vi "Update CD Name Constant.vi"(7 "vi Name":string, 8 "error in":errorcluster, 10 "Custom Device Name":string, 11 "lvlib Path":path) -> (0 "error out":errorcluster)   [LabVIEW 2026, in "NIVS_CDEW_MetaDataObj.lvclass"]
uses:
  NIVS_CDEW_MetaDataObj.lvclass
  NIVS_CDEW_MetaDataObj.lvclass/NIVS_CDEW_MetaDataObj.ctl
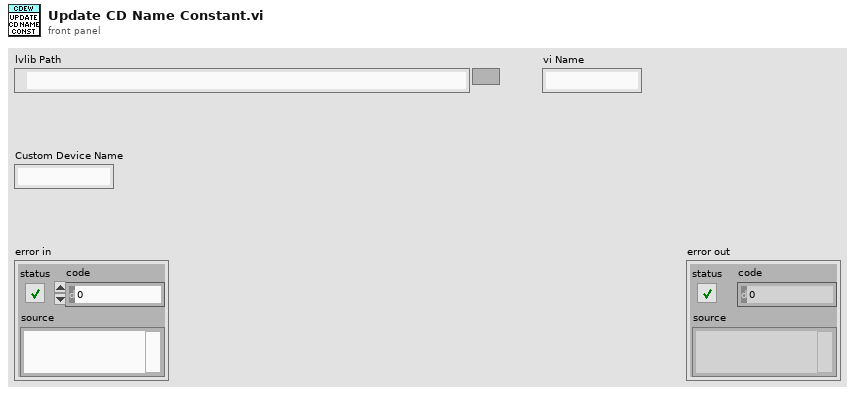
[diagram p1: front panel]
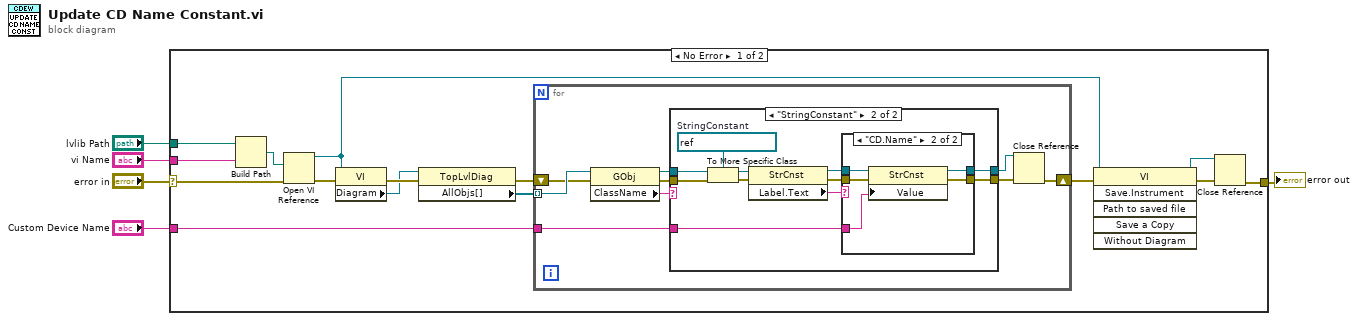
[diagram p0: block diagram]
diagram:
  n1 = case shown="No Error" "error in" {
    selector: "error in" -> [w7 w50]
    tunnel: "lvlib Path" -> [w6 _]
    tunnel: [w19 w50] -> w4
    tunnel: "vi Name" -> [w18 _]
    tunnel: "Custom Device Name" -> [w12 _]
    frame No Error {
      n2 = Build Path(base path=w6, name or relative path=w18) -> (appended path=w20:path)
      n3 = Open VI Reference(vi path=w20, error in (no error)=w7) -> (vi reference=w9:refnum<vi>, error out=w17:errorcluster)  [unwired: 4 in]
      n4 = property class="VI"(reference=w9, error in=w17) -> (error out=w16:errorcluster, "Diagram"=w15:refnum<vi>)  [unwired: 1 out]
      n5 = property class="TopLvlDiag"(reference=w15, error in=w16) -> (error out=w13:errorcluster, "AllObjs[]"=w14:refnum<vi>[])  [unwired: 1 out]
      n6 = for {
        tunnel: w14 -> [w29] mode=indexing
        shift-right: [w23] -> w11
        shift-left: w13 -> [w28]
        tunnel: w12 -> [w21]
        n7 = property class="GObj"(reference=w29, error in=w28) -> (reference out=w25:refnum<vi>, error out=w26:errorcluster, "ClassName"=w27:string)
        n8 = case shown="\"StringConstant\"" w27 {
          tunnel: w26 -> [w31 w42]
          tunnel: w25 -> [w30 w41]
          tunnel: [w31 w34] -> w24
          tunnel: [w30 w33] -> w22
          tunnel: w21 -> [_ w32]
          frame Default {
          }
          frame "StringConstant" {
            w40 = refnum<vi> refnum  # StringConstant
            n9 = To More Specific Class(target class=w40, reference=w41, error in=w42) -> (specific class reference=w38:refnum<vi>, error out=w39:errorcluster)
            n10 = property class="StrCnst"(reference=w38, error in=w39) -> (reference out=w35:refnum<vi>, error out=w36:errorcluster, "Label.Text"=w37:string)
            n11 = case shown="\"CD.Name\"" w37 {
              tunnel: w36 -> [w44 w49]
              tunnel: w35 -> [w43 w48]
              tunnel: [w44 w47] -> w34
              tunnel: [w43 w46] -> w33
              tunnel: w32 -> [_ w45]
              frame Default {
              }
              frame "CD.Name" {
                n12 = property class="StrCnst"(reference=w48, error in=w49, "Value"=w45) -> (reference out=w46:refnum<vi>, error out=w47:errorcluster)
              }
            }
          }
        }
        n13 = Close Reference(reference=w22, error in (no error)=w24) -> (error out=w23:errorcluster)
      }
      n14 = invoke class="VI" method="Save.Instrument"(reference=w9, error in=w11) -> (reference out=w8:refnum<vi>, error out=w10:errorcluster)  [unwired: 4 in, 4 out]
      n15 = Close Reference(reference=w8, error in (no error)=w10) -> (error out=w19:errorcluster)
    }
    frame Error {
    }
  }
  "error out" <- w4
